vi "ICNC Stop Motors All And Clear.vi"(8 "error in (no error)":errorcluster caption="entrée d'erreur (pas d'erreur)") -> (0 "error out":errorcluster caption="sortie d'erreur", 3 "function return":u32)   [LabVIEW 2017, in "ICNC2.lvlib"]
doc: "DWORD ICNC_StopMotorsAllAndClear(void);"
uses:
  ICNC2.lvlib
  <userlib>/ICNC/ICNC2.dll
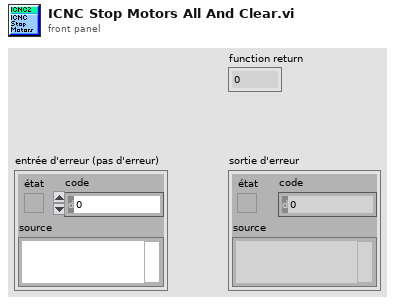
[diagram p1: front panel]
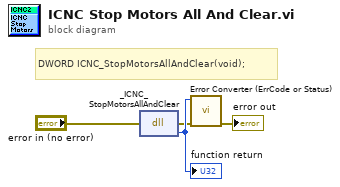
[diagram p0: block diagram]
diagram:
  # "DWORD ICNC_StopMotorsAllAndClear(void);"
  n1 = dll-call lib="C:/Program Files (x86)/National Instruments/LabVIEW 2017/user.lib/ICNC/ICNC2.*" fn="_ICNC_StopMotorsAllAndClear"(error in="error in (no error)") -> (error out=w2:errorcluster, w4:u32)  [unwired: 2 in, 1 out]
  "function return" <- w4
  n2 = call "Error Converter (ErrCode or Status).vi"("error in (no error)"=w2, "error code"=w4) -> ("error out"=→"error out":errorcluster)  [unwired: 9 in]
